vi "BoolToString.vi"(11 "outcome":bool) -> (3 "String":string)   [LabVIEW 2019]
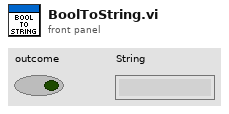
[diagram p1: front panel]
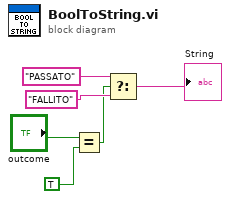
[diagram p0: block diagram]
diagram:
  n1 = Equal?(x="outcome", y=TRUE) -> (x = y?=w3:bool)
  n2 = Select(t="PASSATO", s=w3, f="FALLITO") -> (s? t:f=→"String":string)
